vi "create single value wavelength of desired length.vi"(9 "waveform (with desired single value)":waveform(dbl), 11 "waveform in (for length)":waveform(dbl)) -> (3 "output waveform":waveform(dbl))   [LabVIEW 2025]
uses:
  <vilib>/Waveform/WDTOps.llb/WDT Number of Waveform Samples DBL.vi
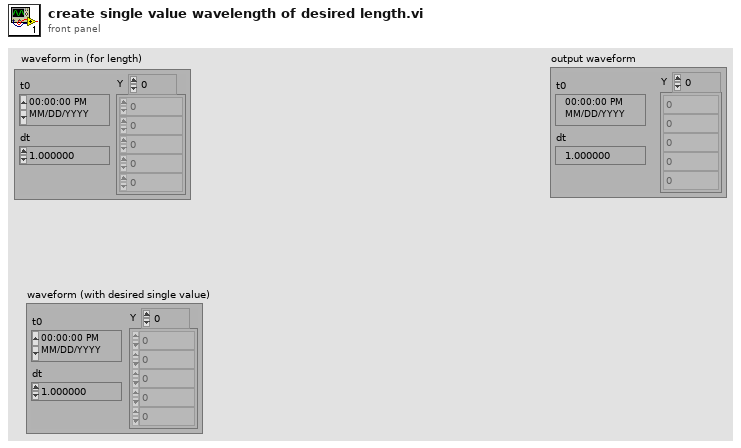
[diagram p1: front panel]
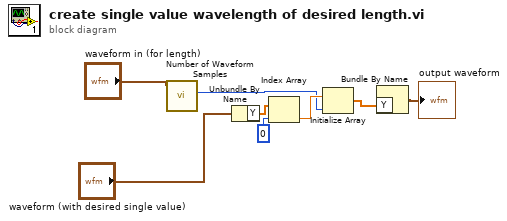
[diagram p0: block diagram]
diagram:
  n1 = call-poly <vilib>:"Number of Waveform Samples.vi"("waveform in"="waveform in (for length)") -> ("number of samples"=w3:i32)  [unwired: 8 in, 2 out]
  n2 = Unbundle By Name("waveform (with desired single value)") -> ("Y"=w8:dbl[])
  n3 = Index Array(array=w8, index=0) -> (element=w6:dbl)
  n4 = Initialize Array(w6, w3) -> (w5:dbl[])
  n5 = Bundle By Name("Y"=w5) -> (→"output waveform":waveform(dbl))  [unwired: 1 in]
